vi "data_retrieval_processing_pipeline.vi"() -> ()   [LabVIEW 2021]
uses:
  a5b8f340-0aaf-3fc0-001e-aaef3e36ac3f.vi
  1634fdf6-5eff-3fe9-09cf-f9bccf8fe73f.vi
panel:
  out "time spent (ms)":u32
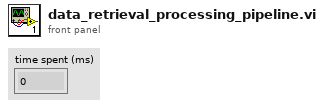
[diagram p1: front panel]
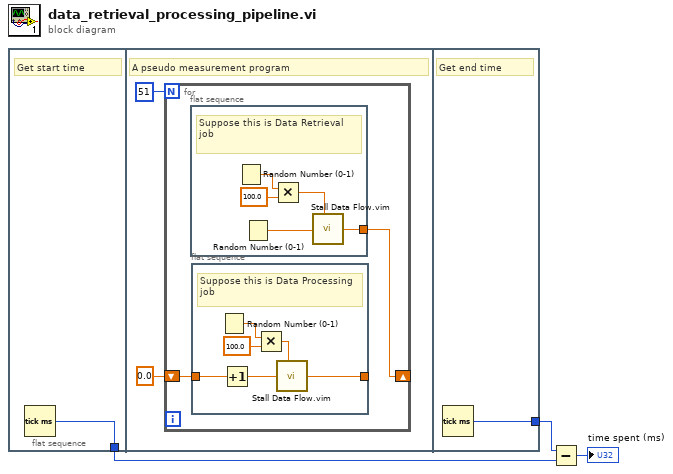
[diagram p0: block diagram]
diagram:
  n1 = flat-sequence {
    tunnel: [w4] -> w2
    tunnel: [w20] -> w3
    frame #0 {
      # "Get start time"
      n2 = Tick Count (ms)() -> (millisecond timer value=w4:u32)
    }
    frame #1 {
      # "A pseudo measurement program"
      n3 = for {
        N: 51 -> [_]
        shift-right: [w8] -> _
        shift-left: 0.0 -> [w7]
        n4 = flat-sequence {
          tunnel: [w19] -> w8
          frame #0 {
            # "Suppose this is Data Retrieval job"
            n5 = Random Number (0-1)() -> (number: 0 to 1=w18:dbl)
            n6 = Random Number (0-1)() -> (number: 0 to 1=w15:dbl)
            n7 = Multiply(x=w18, y=100.0) -> (x*y=w16:dbl)
            n8 = call "Stall Data Flow.vim"("value in"=w15, "milliseconds to wait"=w16) -> ("value out"=w19:dbl)  [unwired: 1 out]
          }
        }
        n9 = flat-sequence {
          tunnel: w7 -> [w10]
          tunnel: [w14] -> _
          frame #0 {
            # "Suppose this is Data Processing job"
            n10 = Random Number (0-1)() -> (number: 0 to 1=w12:dbl)
            n11 = Increment(x=w10) -> (x+1=w9:dbl)
            n12 = Multiply(x=w12, y=100.0) -> (x*y=w11:dbl)
            n13 = call "Stall Data Flow.vim"("value in"=w9, "milliseconds to wait"=w11) -> ("value out"=w14:dbl)  [unwired: 1 out]
          }
        }
      }
    }
    frame #2 {
      # "Get end time"
      n14 = Tick Count (ms)() -> (millisecond timer value=w20:u32)
    }
  }
  n15 = Subtract(x=w3, y=w2) -> (x-y=→"time spent (ms)":u32)
